vi "CheckAll-Quit.vi"() -> (1 "All-Quit":bool)   [LabVIEW 2019]
uses:
  Globals and TypeDefs/gGeneral.vi
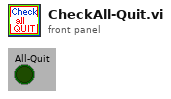
[diagram p1: front panel]
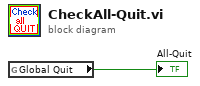
[diagram p0: block diagram]
diagram:
  n1 = global read "gGeneral.vi" "Global Quit"() -> (→"All-Quit":bool)
